vi "Test Read InteropAssembly Ref.vi"() -> ()   [LabVIEW 2020]
uses:
  C:/Users/dzoni/Documents/NJ/Playground/LV/TCP Client/client/builds/ClientApp1/ClientApp1.dll
  builds/ClientApp1/ClientApp1.dll
panel:
  in  "Constructor Selection":T1(ring)=enum."Constructor Ptr"
  out "Size":i32
  out "Size 1":i32
  out "IsValid":bool
  out "ID":string
  out "Port":u16
  out "Data 2":string
  out "Data":string
  out "Address":string
  out "error out":errorcluster
  # "Error 1172 occurred at Invoke Node \nA .NET exception occurred in an external assembly."
  # "ErrorCode = 56 \nErrorSource = TCP Open Connection\n56 - The network operation exceeded \nthe user-specified or system time limit."
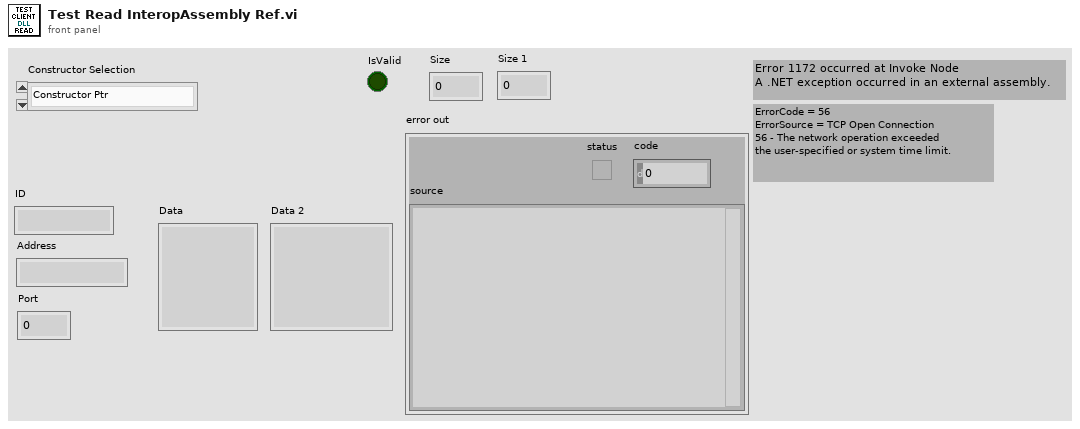
[diagram p1: front panel]
types:
  T1 = enum16{"No Constructor (GetRef)", "Constructor new", "Constructor Ptr"}
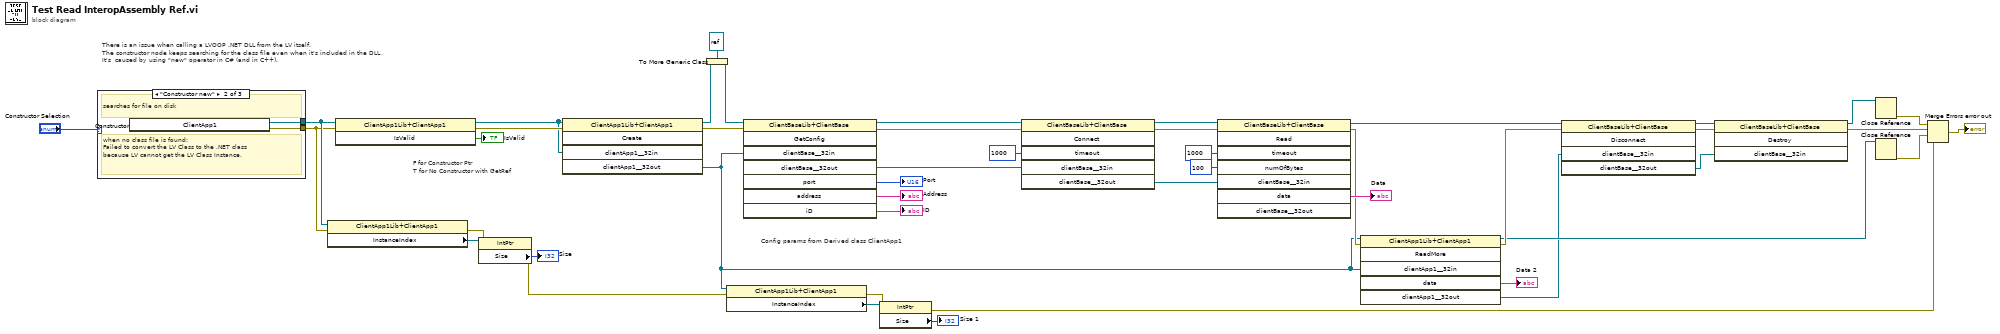
[diagram p0: block diagram]
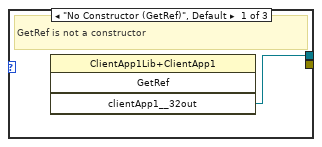
[diagram p2: hidden frame]
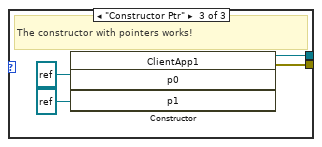
[diagram p3: hidden frame]
diagram:
  # "Config params from Derived class ClientApp1"
  # "F for Constructor Ptr\nT for No Constructor with GetRef"
  # "There is an issue when calling a LVOOP .NET DLL from the LV itself.\nThe constructor node keeps searching for the class file even when it's included in the DLL.\nIt's  caused by using \"new\" operator in C# (and in C++)."
  n1 = case shown="\"Constructor new\"" "Constructor Selection" {
    tunnel: [_ w48 w53] -> w6
    tunnel: [w47 w49 w52] -> w12
    frame "No Constructor (GetRef)", Default {
      # "GetRef is not a constructor"
      n2 = invoke class="ClientApp1Lib+ClientApp1" method="GetRef"() -> ("clientApp1__32out"=w47:refnum<k24>)  [unwired: 4 in, 3 out]
    }
    frame "Constructor new" {
      # "when no class file is found:\nFailed to convert the LV Class to the .NET class \nbecause LV cannot get the LV Class Instance."
      # "searches for file on disk"
      n3 = constructor class="ClientApp1Lib+ClientApp1"() -> (reference out=w49:refnum<k24>, error out=w48:errorcluster)  [unwired: 3 in, 1 out]
    }
    frame "Constructor Ptr" {
      # "The constructor with pointers works!"
      n4 = constructor class="ClientApp1Lib+ClientApp1"("p0"=refnum<k24> refnum, "p1"=refnum<k24> refnum) -> (reference out=w52:refnum<k24>, error out=w53:errorcluster)  [unwired: 3 in, 3 out]
    }
  }
  n5 = property class="ClientApp1Lib+ClientApp1"(reference=w12, error in=w6) -> (error out=w5:errorcluster, "InstanceIndex"=w9:refnum<k24>)  [unwired: 1 out]
  n6 = invoke class="ClientApp1Lib+ClientApp1" method="IsValid"(reference=w12, error in=w6) -> (reference out=w14:refnum<k24>, error out=w15:errorcluster, "IsValid"=→"IsValid":bool)  [unwired: 1 in]
  n7 = property class="IntPtr"(reference=w9, error in=w5) -> (error out=w2:errorcluster, "Size"=→"Size":i32)  [unwired: 1 out]
  n8 = invoke class="ClientApp1Lib+ClientApp1" method="Create"(reference=w14, error in=w15, "clientApp1__32in"=w14) -> (reference out=w20:refnum<k24>, error out=w4:errorcluster, "clientApp1__32out"=w13:refnum<k24>)  [unwired: 2 in, 2 out]
  n9 = To More Generic Class(target class=refnum<k24> refnum, reference=w20) -> (generic class reference=w19:refnum<k24>)
  n10 = property class="ClientApp1Lib+ClientApp1"(reference=w13, error in=w2) -> (error out=w3:errorcluster, "InstanceIndex"=w11:refnum<k24>)  [unwired: 1 out]
  n11 = invoke class="ClientBaseLib+ClientBase" method="GetConfig"(reference=w19, error in=w4, "clientBase__32in"=w13) -> (reference out=w43:refnum<k24>, error out=w41:errorcluster, "clientBase__32out"=w42:refnum<k24>, "port"=→"Port":u16, "address"=→"Address":string, "iD"=→"ID":string)  [unwired: 5 in, 2 out]
  n12 = property class="IntPtr"(reference=w11, error in=w3) -> (error out=w1:errorcluster, "Size"=→"Size 1":i32)  [unwired: 1 out]
  n13 = invoke class="ClientBaseLib+ClientBase" method="Connect"(reference=w43, error in=w41, "timeout"=1000, "clientBase__32in"=w42) -> (reference out=w39:refnum<k24>, error out=w38:errorcluster, "clientBase__32out"=w35:refnum<k24>)  [unwired: 2 in, 3 out]
  n14 = invoke class="ClientBaseLib+ClientBase" method="Read"(reference=w39, error in=w38, "timeout"=1000, "numOfBytes"=100, "clientBase__32in"=w35) -> (reference out=w31:refnum<k24>, error out=w33:errorcluster, "data"=→"Data":string)  [unwired: 3 in, 5 out]
  n15 = invoke class="ClientApp1Lib+ClientApp1" method="ReadMore"(reference=w13, error in=w33, "clientApp1__32in"=w13) -> (reference out=w25:refnum<k24>, error out=w30:errorcluster, "data"=→"Data 2":string, "clientApp1__32out"=w17:refnum<k24>)  [unwired: 3 in, 2 out]
  n16 = invoke class="ClientBaseLib+ClientBase" method="Disconnect"(reference=w31, error in=w30, "clientBase__32in"=w17) -> (reference out=w27:refnum<k24>, error out=w28:errorcluster, "clientBase__32out"=w29:refnum<k24>)  [unwired: 2 in, 2 out]
  n17 = invoke class="ClientBaseLib+ClientBase" method="Destroy"(reference=w27, error in=w28, "clientBase__32in"=w29) -> (reference out=w26:refnum<k24>, error out=w24:errorcluster)  [unwired: 1 in, 2 out]
  n18 = Close Reference(reference=w26) -> (error out=w22:errorcluster)  [unwired: 1 in]
  n19 = Close Reference(reference=w25) -> (error out=w21:errorcluster)  [unwired: 1 in]
  n20 = Merge Errors(w22, w24, w21, w1) -> (→"error out":errorcluster)
